vi "timetest8.vi"() -> ()   [LabVIEW 2015]
uses:
  BERTTA.dll
panel:
  in  "pause":i32
  in  "elapsed":i32
  in  "Tcurrent":dbl
  out "setpoint":dbl
  in  "enable":i32
  in  "Tinit":dbl
  in  "Tset":dbl
  in  "ramp_time":i32
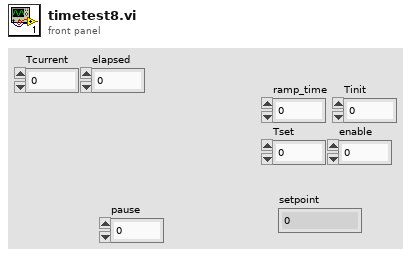
[diagram p1: front panel]
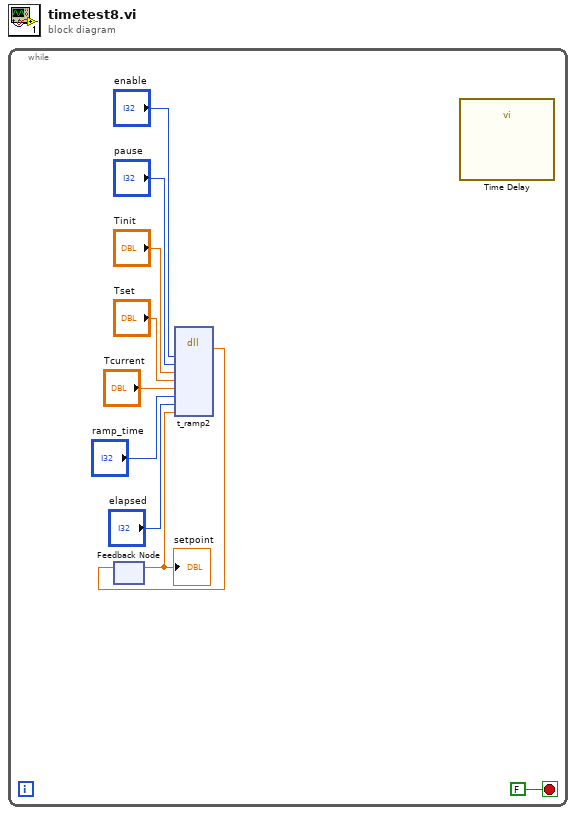
[diagram p0: block diagram]
diagram:
  n1 = while {
    stop <- FALSE stop-if-true
    n2 = feedback #1() -> (w2:dbl)  [unwired: 1 in]
    "setpoint" <- w2
    n3 = dll-call lib="C:/Users/xlaraser/Documents/Visual Studio 2017/Projects/Bertta/BERTTA/Debug/BERTTA.dll" fn="t_ramp2"("enable"="enable", "pause"="pause", "Tinit"="Tinit", "Tset"="Tset", "Tcurrent"="Tcurrent", "ramp_time"="ramp_time", "elapsed"="elapsed", "sp_old"=w2) -> ("return type"=w3:dbl)  [unwired: 11 in, 2 out]
    n4 = feedback-in #1(w3) -> ()
    n5 = call "Time Delay"() -> ()  [unwired: 11 in, 1 out]
  }
